vi "AddItem.vi"(8 "error in (no error)":errorcluster caption="错误输入（无错误）", 11 "DigitalDisplay 输入":refnum<class "DigitalDisplay.lvclass">) -> (0 "error out":errorcluster caption="错误输出", 3 "DigitalDisplay 输出":refnum<class "DigitalDisplay.lvclass">)   [LabVIEW 2018, in "DataDisplay.lvlib" / "DigitalDisplay.lvclass"]
uses:
  DigitalDisplay.lvclass
  DigitalDisplay.lvclass/DigitalDisplay.ctl
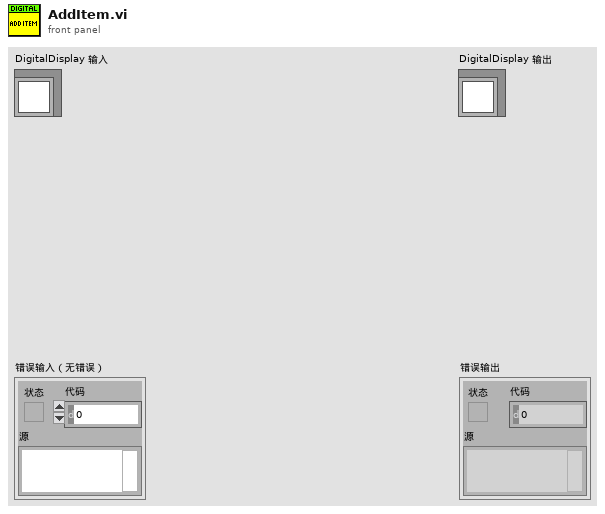
[diagram p1: front panel]
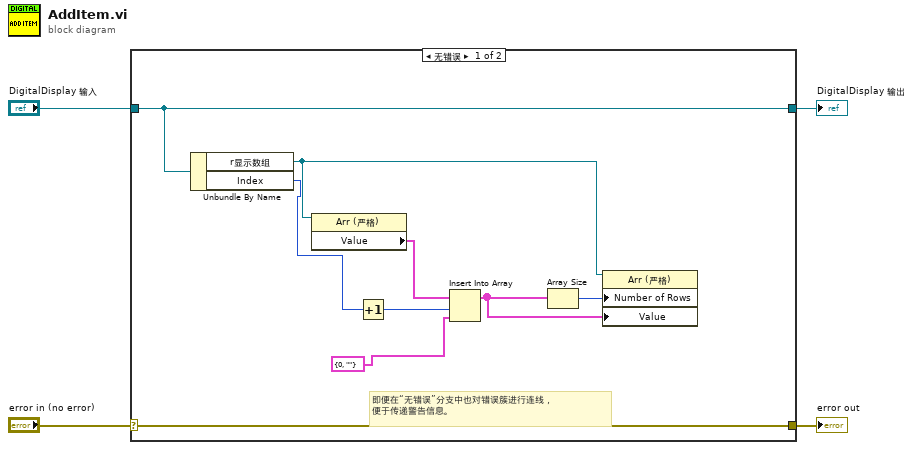
[diagram p0: block diagram]
diagram:
  n1 = case shown="无错误" "error in (no error)" {
    selector: "error in (no error)" -> [w13 w15]
    tunnel: [w13 w15] -> w3
    tunnel: [w9 w14] -> w1
    tunnel: "DigitalDisplay 输入" -> [w9 w14]
    frame No Error {
      # "即便在“无错误”分支中也对错误簇进行连线，\n便于传递警告信息。"
      n2 = Unbundle By Name(w9) -> ("r显示数组"=w8:refnum<vi>, "Index"=w5:i32)
      n3 = property class="Arr (严格)"(reference=w8) -> ("Value"=w7:cluster{"通道选择":u16, "数值":string}[])  [unwired: 1 in, 2 out]
      n4 = Increment(x=w5) -> (x+1=w10:i32)
      n5 = Insert Into Array(array=w7, index=w10, new element=cluster{"通道选择":u16, "数值":string} {"通道选择"=0, "数值"=""} ("簇")) -> (w11:cluster{"通道选择":u16, "数值":string}[])
      n6 = Array Size(array=w11) -> (size(s)=w12:i32)
      n7 = property class="Arr (严格)"(reference=w8, "Number of Rows"=w12, "Value"=w11) -> ()  [unwired: 1 in, 2 out]
    }
    frame Error {
    }
  }
  "error out" <- w3
  "DigitalDisplay 输出" <- w1
